vi "CANOpen_Main_Close HB NG EM.vi"(8 "error in (no error)":errorcluster, 10 "Security Ref":T1, 11 "interface object":refnum<k20>) -> (0 "error out":errorcluster)   [LabVIEW 2021, in "CANOpen Addon Engine.lvlib"]
uses:
  CANOpen Addon Engine.lvlib
  CANOpen_HB_NG_EM Refs.ctl
  <vilib>/CANopenLib/CANOPEN.llb/CANopen SDO Create.vi
  <vilib>/CANopenLib/CANOPEN.llb/CANopen SDO Write [U16].vi
  <vilib>/CANopenLib/CANOPEN.llb/CANopen SDO Close.vi
  <vilib>/CANopenLib/CANOPEN.llb/CANopen Heartbeat Close.vi
  <vilib>/CANopenLib/CANOPEN.llb/CANopen SDO Write [U8].vi
  <vilib>/CANopenLib/CANOPEN.llb/CANopen Node Guarding Close.vi
  <vilib>/CANopenLib/CANOPEN.llb/CANopen Emergency Close.vi
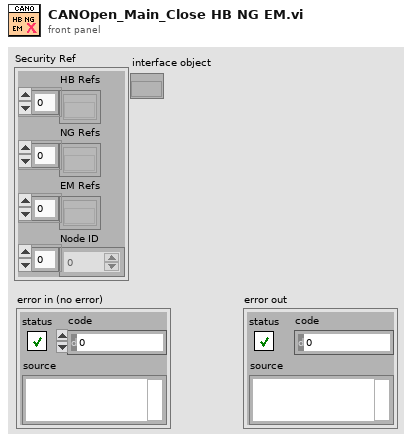
[diagram p1: front panel]
types:
  T1 = typedef "CANOpen Addon Engine.lvlib/CANOpen_HB_NG_EM Refs.ctl" = cluster{"HB Refs":refnum<k20>[], "NG Refs":refnum<k20>[], "EM Refs":refnum<k20>[], "Node ID":u8[]}
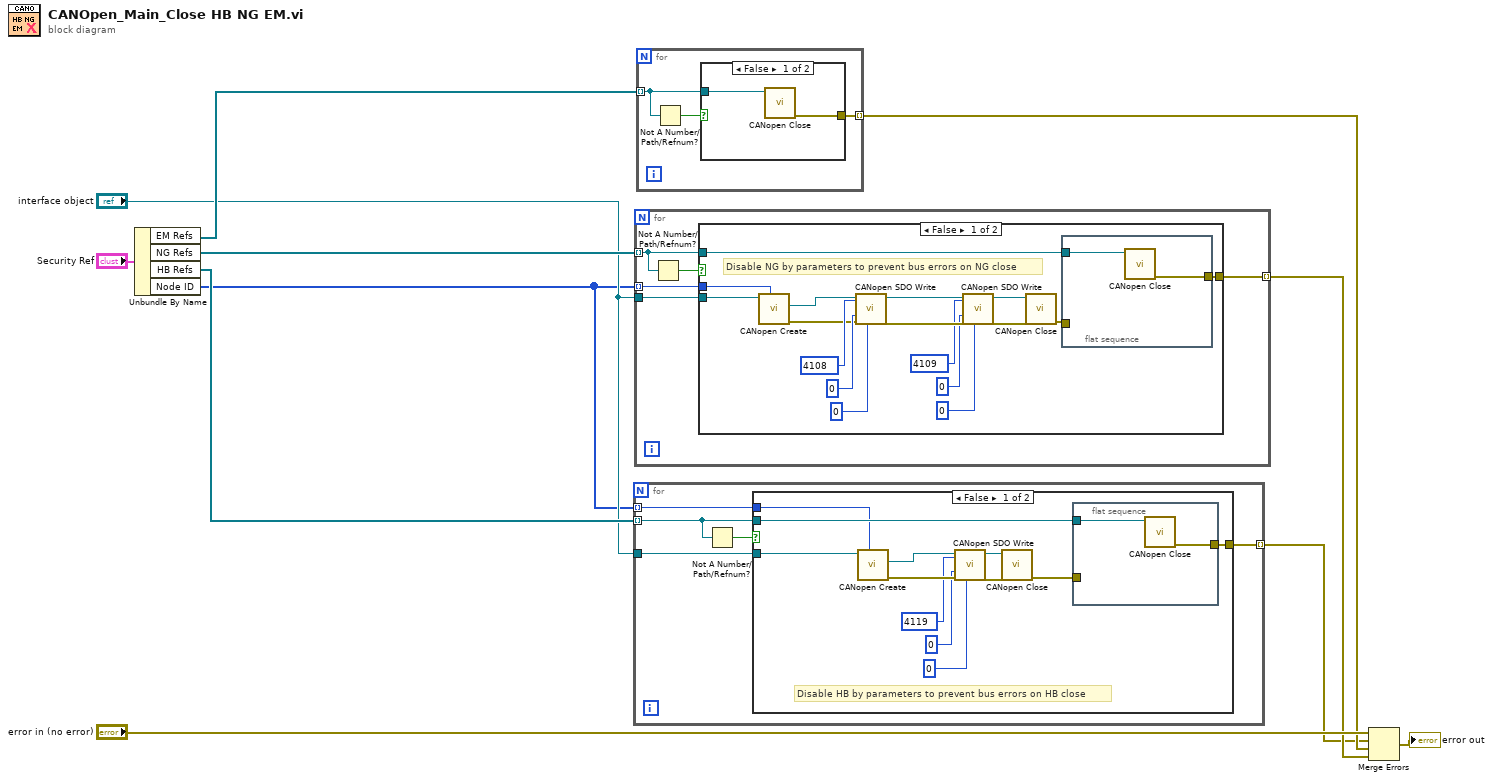
[diagram p0: block diagram]
diagram:
  n1 = Unbundle By Name("Security Ref") -> ("EM Refs"=w6:refnum<k20>[], "NG Refs"=w7:refnum<k20>[], "HB Refs"=w8:refnum<k20>[], "Node ID"=w1:u8[])
  n2 = for {
    tunnel: w8 -> [w15] mode=indexing
    tunnel: [w16] -> w3 mode=indexing
    tunnel: "interface object" -> [w13]
    tunnel: w1 -> [w12] mode=indexing
    n3 = Not A Number/Path/Refnum?(number/path/refnum=w15) -> (NaN/Path/Refnum?=w14:bool)
    n4 = case shown="False" w14 {
      tunnel: w15 -> [w27 _]
      tunnel: [w28 _] -> w16
      tunnel: w13 -> [w19 _]
      tunnel: w12 -> [w18 _]
      frame False {
        # "Disable HB by parameters to prevent bus errors on HB close"
        n5 = call-poly <vilib>:"CANopen Create.vi"("node-ID"=w18, "interface object in"=w19) -> ("error out"=w22:errorcluster, "SDO object out"=w25:refnum<k20>)  [unwired: 7 in, 1 out]
        n6 = call-poly <vilib>:"CANopen SDO Write.vi"("U16 data"=u16 0, "error in (no error)"=w22, "object sub-index (0)"=u8 0, "object index"=u16 4119, "SDO object in"=w25) -> ("error out"=w24:errorcluster, "SDO object out"=w23:refnum<k20>)  [unwired: 4 in, 1 out]
        n7 = call-poly <vilib>:"CANopen Close.vi"("error in (no error)"=w24, "SDO object in"=w23) -> ("error out"=w17:errorcluster)  [unwired: 9 in]
        n8 = flat-sequence {
          tunnel: [w30] -> w28
          tunnel: w27 -> [w29]
          tunnel: w17 -> [_]
          frame #0 {
            n9 = call-poly <vilib>:"CANopen Close.vi"("heartbeat object in"=w29) -> ("error out"=w30:errorcluster)  [unwired: 10 in]
          }
        }
      }
      frame True {
      }
    }
  }
  n10 = for {
    tunnel: w7 -> [w34] mode=indexing
    tunnel: [w35] -> w4 mode=indexing
    tunnel: w1 -> [w32] mode=indexing
    tunnel: "interface object" -> [w31]
    n11 = Not A Number/Path/Refnum?(number/path/refnum=w34) -> (NaN/Path/Refnum?=w33:bool)
    n12 = case shown="False" w33 {
      tunnel: w34 -> [w37 _]
      tunnel: [w52 _] -> w35
      tunnel: w32 -> [w38 _]
      tunnel: w31 -> [w39 _]
      frame False {
        # "Disable NG by parameters to prevent bus errors on NG close"
        n13 = call-poly <vilib>:"CANopen Create.vi"("node-ID"=w38, "interface object in"=w39) -> ("error out"=w41:errorcluster, "SDO object out"=w40:refnum<k20>)  [unwired: 7 in, 1 out]
        n14 = call-poly <vilib>:"CANopen SDO Write.vi"("U16 data"=u16 0 ("Guard Time (ms)"), "error in (no error)"=w41, "object sub-index (0)"=u8 0, "object index"=u16 4108, "SDO object in"=w40) -> ("error out"=w48:errorcluster, "SDO object out"=w46:refnum<k20>)  [unwired: 4 in, 1 out]
        n15 = call-poly <vilib>:"CANopen SDO Write.vi"("U8 data"=u8 0, "error in (no error)"=w48, "object sub-index (0)"=u8 0, "object index"=u16 4109, "SDO object in"=w46) -> ("error out"=w49:errorcluster, "SDO object out"=w47:refnum<k20>)  [unwired: 4 in, 1 out]
        n16 = call-poly <vilib>:"CANopen Close.vi"("error in (no error)"=w49, "SDO object in"=w47) -> ("error out"=w36:errorcluster)  [unwired: 9 in]
        n17 = flat-sequence {
          tunnel: [w54] -> w52
          tunnel: w37 -> [w53]
          tunnel: w36 -> [_]
          frame #0 {
            n18 = call-poly <vilib>:"CANopen Close.vi"("node guarding object in"=w53) -> ("error out"=w54:errorcluster)  [unwired: 10 in]
          }
        }
      }
      frame True {
      }
    }
  }
  n19 = for {
    tunnel: w6 -> [w56] mode=indexing
    tunnel: [w57] -> w5 mode=indexing
    n20 = Not A Number/Path/Refnum?(number/path/refnum=w56) -> (NaN/Path/Refnum?=w55:bool)
    n21 = case shown="False" w55 {
      tunnel: w56 -> [w58 _]
      tunnel: [w59 _] -> w57
      frame False {
        n22 = call-poly <vilib>:"CANopen Close.vi"("emergency object in"=w58) -> ("error out"=w59:errorcluster)  [unwired: 10 in]
      }
      frame True {
      }
    }
  }
  n23 = Merge Errors("error in (no error)", w3, w5, w4) -> (→"error out":errorcluster)
